vi "Harmonic Distortion Analyzer 1 Chan.vi"(6 "advanced search":T4={"approx freq. (optional)"=-1.0, "search (+/- % of Fsampl.)"=5.0} {"search (+/- % of Fsampl.)" format="%0.2p"; "approx freq. (optional)" format="%0.2p"}, 7 "stop search at Nyquist":bool=TRUE, 8 "error in (no error)":errorcluster, 9 "highest harmonic":i32=19, 10 "export mode":T2(ring), 11 "signal in":waveform(dbl)) -> (0 "error out":errorcluster, 1 "components level":dbl[](array[numeric]) format="%.2p", 2 "THD":dbl format="%.2p", 3 "detected fundamental frequency":dbl format="%.2p", 4 "measurement info":T3={"uncertainty"=0.0, "Warning"=FALSE, "comments"="reserved for future use"} {"uncertainty" format="%0.2p"}, 5 "exported signals":T1 {"exported spectrum (dB)"."dB Spectrum (Hann)" format="%.2p"; "exported spectrum (dB)"."df" format="%.2p"; "exported spectrum (dB)"."f0" format="%.2p"})   [LabVIEW 2020, in "NI_MAPro.lvlib"]
doc: "Takes a signal in and performs a full harmonic analysis, including measuring the fundamental frequency tone and harmonics, and returning the fundamental frequency, all harmonic amplitude levels, and the total harmonic distortion (THD). Wire data to the <B>signal in</B> input to determine the polymorphic instance to use or manually select the instance."
uses:
  NI_MAPro.lvlib
  NI_MABase.lvlib
panel:
  in  "Nyquist message":string="Highest harmonic limited by Nyquist to "
  # "Harmonic Distortion\nAnalyzer"
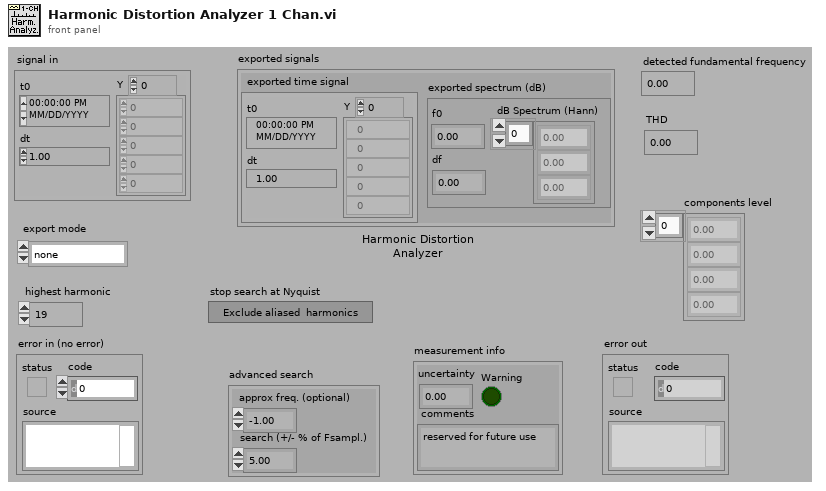
[diagram p1: front panel]
types:
  T1 = cluster{"exported time signal":waveform(dbl), "exported spectrum (dB)":cluster{"f0":dbl, "df":dbl, "dB Spectrum (Hann)":dbl[]}}
  T2 = enum16{"none", "input signal", "fundamental signal", "residual signal", "harmonics only", "noise and spurs"}
  T3 = cluster{"uncertainty":dbl, "Warning":bool, "comments":string}
  T4 = cluster{"approx freq. (optional)":dbl, "search (+/- % of Fsampl.)":dbl}
  T5 = enum16{"none", "input signal", "detected signal", "residual signal"}
  T6 = cluster{"aliased tone frequency":dbl, "search (+/- % of Fsampl.)":dbl}
  T7 = cluster{"signal in":waveform(dbl), cluster{dbl, dbl, dbl[]}}
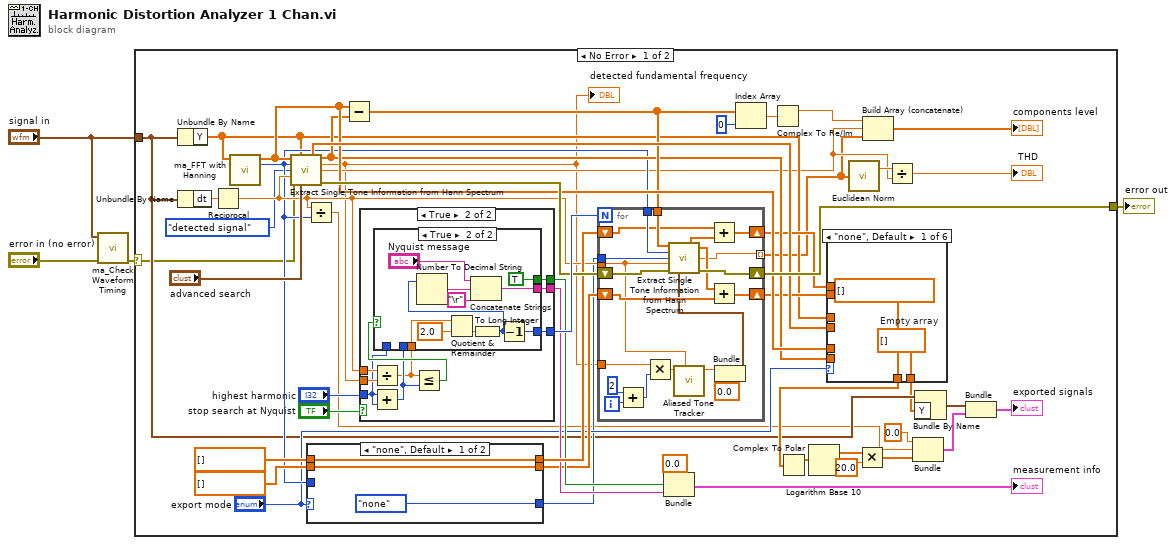
[diagram p0: block diagram]
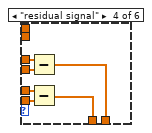
[diagram p4: hidden frame]
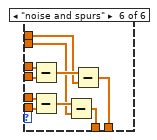
[diagram p6: hidden frame]
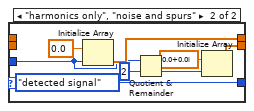
[diagram p7: hidden frame]
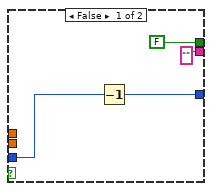
[diagram p8: hidden frame]
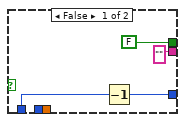
[diagram p9: hidden frame]
diagram:
  n1 = call "ma_Check Waveform Timing.vi"("error in (no error)"="error in (no error)", "signal in"="signal in") -> ("error out"=w3:errorcluster)  [unwired: 1 in, 8 out]
  n2 = case shown="No Error" w3 {
    selector: w3 -> [w5 w137]
    tunnel: [w43 w137] -> w4
    tunnel: "signal in" -> [w16 _]
    frame No Error {
      n3 = Unbundle By Name(w16) -> ("Y"=w17:dbl[])
      n4 = Unbundle By Name(w16) -> ("dt"=w18:dbl)
      n5 = Reciprocal(x=w18) -> (1/x=w26:dbl)
      n6 = call "ma_FFT with Hanning.vi"("time signal data"=w17) -> ("FFT size"=w25:i32, "complex Hann spectrum"=w37:cdb[])  [unwired: 2 in, 7 out]
      n7 = call "Extract Single Tone Information from Hann Spectrum.vi"("complex spectrum in"=w37, "time signal in"=w17, "FFT size"=w25, "export mode"=T5."detected signal" ("exported time signal"), "sampling frequency"=w26, "error in"=w5, "advanced search"="advanced search") -> ("time signal out"=w38:dbl[], "complex spectrum out"=w35:cdb[], "detected frequency"=w6:dbl, "detected amplitude"=w10:dbl, "error out"=w50:errorcluster)  [unwired: 4 out]
      "detected fundamental frequency" <- w6
      n8 = Divide(x=w26, y=w25) -> (x/y=w13:dbl)
      n9 = case shown="\"none\", Default" "export mode" {
        tunnel: [T5."none" ("Bundle Element") T5."detected signal" ("Bundle Element")] -> w19
        tunnel: [w79 w87] -> w48
        tunnel: w25 -> [_ w83]
        tunnel: dbl[] [] -> [w79 _]
        tunnel: [w78 w81] -> w32
        tunnel: cdb[] [] -> [w78 _]
        frame "none", Default {
        }
        frame "harmonics only", "noise and spurs" {
          n10 = Initialize Array(0.0 ("Element Data"), w83) -> (w87:dbl[])
          n11 = Quotient & Remainder(x=w83, y=2) -> (floor(x/y)=w84:i32)  [unwired: 1 out]
          n12 = Initialize Array(cdb 0.0+0.0i ("Element Data"), w84) -> (w81:cdb[])
        }
      }
      n13 = Subtract(x=w37, y=w35) -> (x-y=w36:cdb[])
      n14 = case shown="True" "stop search at Nyquist" {
        tunnel: w26 -> [_ w122]
        tunnel: w6 -> [_ w121]
        tunnel: "highest harmonic" -> [w113 w114]
        tunnel: [w110 w117] -> w51
        tunnel: ["" w116] -> w41
        tunnel: [FALSE w115] -> w42
        frame False {
          n15 = Decrement(x=w113) -> (x-1=w110:i32)
        }
        frame True {
          n16 = Divide(x=w122, y=w121) -> (x/y=w118:dbl)
          n17 = Add(x=w114, y=w114) -> (x+y=w119:i32)
          n18 = Less Or Equal?(x=w118, y=w119) -> (x <= y?=w120:bool)
          n19 = case shown="True" w120 {
            tunnel: w119 -> [_ _]
            tunnel: w118 -> [_ w135]
            tunnel: [w124 w129] -> w117
            tunnel: ["" w131] -> w116
            tunnel: [FALSE TRUE] -> w115
            tunnel: w114 -> [w123 _]
            frame False {
              n20 = Decrement(x=w123) -> (x-1=w124:i32)
            }
            frame True {
              n21 = Quotient & Remainder(x=w135, y=2.0) -> (floor(x/y)=w134:dbl)  [unwired: 1 out]
              n22 = To Long Integer(number=w134) -> (32bit integer=w128:i32)
              n23 = Number To Decimal String(number=w128) -> (decimal integer string=w133:string)  [unwired: 1 out]
              n24 = Concatenate Strings("Nyquist message", w133, "\r") -> (w131:string)
              n25 = Decrement(x=w128) -> (x-1=w129:i32)
            }
          }
        }
      }
      n26 = for {
        N: w51 -> [_]
        tunnel: w36 -> [w108]
        tunnel: w6 -> [w109]
        tunnel: w25 -> [w107]
        tunnel: w26 -> [w93]
        shift-right: [w103] -> w43
        shift-left: w50 -> [w106]
        tunnel: [w94] -> w9 mode=indexing
        shift-right: [w104] -> w34
        shift-left: w48 -> [w98]
        shift-right: [w97] -> w33
        shift-left: w32 -> [w96]
        tunnel: w19 -> [w91]
        i -> [w102]
        n27 = Add(x=2, y=w102) -> (x+y=w100:i32)
        n28 = Multiply(x=w109, y=w100) -> (x*y=w105:dbl)
        n29 = call "Aliased Tone Tracker.vi"("sampling frequency"=w93, "real tone frequency"=w105) -> ("aliased tone frequency"=w89:dbl)  [unwired: 1 in, 8 out]
        n30 = Bundle("aliased tone frequency"=w89, "search (+/- % of Fsampl.)"=0.0) -> (w92:T6)  [unwired: 1 out]
        n31 = call "Extract Single Tone Information from Hann Spectrum.vi"("complex spectrum in"=w108, "FFT size"=w107, "export mode"=w91, "sampling frequency"=w93, "error in"=w106, "advanced search"=w92) -> ("time signal out"=w99:dbl[], "complex spectrum out"=w95:cdb[], "detected amplitude"=w94:dbl, "error out"=w103:errorcluster)  [unwired: 1 in, 5 out]
        n32 = Add(x=w98, y=w99) -> (x+y=w104:dbl[])
        n33 = Add(x=w95, y=w96) -> (x+y=w97:cdb[])
      }
      n34 = Bundle(0.0, w42, w41) -> (→"measurement info":cluster{dbl, bool, string})  [unwired: 1 out]
      n35 = Index Array(array=w36, index=0 ("Index")) -> (element=w47:cdb)
      n36 = Complex To Re/Im(x + iy=w47) -> (x=w7:dbl)  [unwired: 1 out]
      n37 = case shown="\"none\", Default" "export mode" {
        tunnel: [w55 w57 w59 w63 w67 w69] -> w15
        tunnel: w37 -> [_ w56 _ w62 _ w72]
        tunnel: w38 -> [_ _ w59 w64 _ w73]
        tunnel: [cdb[] [] ("dB Spectrum (Hann)") w56 w58 w60 w66 w68] -> w30
        tunnel: w17 -> [_ w57 _ w65 _ w74]
        tunnel: w35 -> [_ _ w58 w61 _ w71]
        tunnel: w34 -> [_ _ _ _ w67 w75]
        tunnel: w33 -> [_ _ _ _ w66 w70]
        frame "none", Default {
          w55 = dbl[] []  # Empty array
        }
        frame "input signal" {
        }
        frame "fundamental signal" {
        }
        frame "residual signal" {
          n38 = Subtract(x=w65, y=w64) -> (x-y=w63:dbl[])
          n39 = Subtract(x=w62, y=w61) -> (x-y=w60:cdb[])
        }
        frame "harmonics only" {
        }
        frame "noise and spurs" {
          n40 = Subtract(x=w74, y=w73) -> (x-y=w77:dbl[])
          n41 = Subtract(x=w72, y=w71) -> (x-y=w76:cdb[])
          n42 = Subtract(x=w76, y=w70) -> (x-y=w68:cdb[])
          n43 = Subtract(x=w77, y=w75) -> (x-y=w69:dbl[])
        }
      }
      n44 = Complex To Polar(r * e^(i*theta)=w30) -> (r=w29:dbl[])  [unwired: 1 out]
      n45 = Logarithm Base 10(1:w29) -> (0:w28:dbl[])
      n46 = call "Euclidean Norm.vi"("X"=w9) -> ("root square value"=w45:dbl)  [unwired: 1 out]
      n47 = Multiply(x=w28, y=20.0) -> (x*y=w12:dbl[])
      n48 = Build Array (concatenate)(w7, w10, w9) -> (→"components level":dbl[])
      n49 = Divide(x=w45, y=w10) -> (x/y=→"THD":dbl)
      n50 = Bundle(0.0, w13, w12) -> (w11:cluster{dbl, dbl, dbl[]})  [unwired: 1 out]
      n51 = Bundle By Name(cluster=w16, "Y"=w15) -> (w21:waveform(dbl))
      n52 = Bundle("signal in"=w21, w11) -> (→"exported signals":T7)  [unwired: 1 out]
    }
    frame Error {
    }
  }
  "error out" <- w4
